vi "BotSpeak_Variables.vi"(1 "Scaling":T1(array[cluster])=[{"upper limit"=0.0, "lower limit"=0.0, "scale"=1.0}, {"upper limit"=0.0, "lower limit"=0.0, "scale"=1.0}, {"upper limit"=0.0, "lower limit"=0.0, "scale"=1.0}, {"upper limit"=0.0, "lower limit"=0.0, "scale"=1.0}, {"upper limit"=0.0, "lower limit"=0.0, "scale"=1.0}, {"upper limit"=0.0, "lower limit"=0.0, "scale"=1.0}, {"upper limit"=0.0, "lower limit"=0.0, "scale"=1.0}, {"upper limit"=0.0, "lower limit"=0.0, "scale"=1.0}, {"upper limit"=0.0, "lower limit"=0.0, "scale"=1.0}, {"upper limit"=0.0, "lower limit"=0.0, "scale"=1.0}, {"upper limit"=0.0, "lower limit"=0.0, "scale"=1.0}], 2 "Var #?":bool[](array[boolean])=[TRUE, TRUE, TRUE, TRUE, TRUE, TRUE, TRUE, TRUE, TRUE, TRUE, TRUE], 3 "Variables":string[](array[string])) -> (0 "Binary out":u8[](array[numeric]) format="%.0x")   [LabVIEW 2014]
panel:
  out "Vars":string[](array[string])
  # "Variable # or Value of Variable"
  # "sources:\n\n200 (C8) - TMR[#]\n201 (C9) - AI[#]\n202 (CA) - DIO[#]\n203 (CB) - PWM[#]\n204 (CC) - SERVO[#]\n205 (CD) - VAR[#]\n\n220 (DC) - TMR[var]\n221 (DD) - AI[var]\n222 (DE) - DIO[var]\n223 (DF) - PWM[var]\n224 (E0) - SERVO[var]\n225 (E1) - VAR[var]\n\n252 (FC) - \n253 (FD) - var[var]\n254 (FE) - \n255 (FF) - var#"
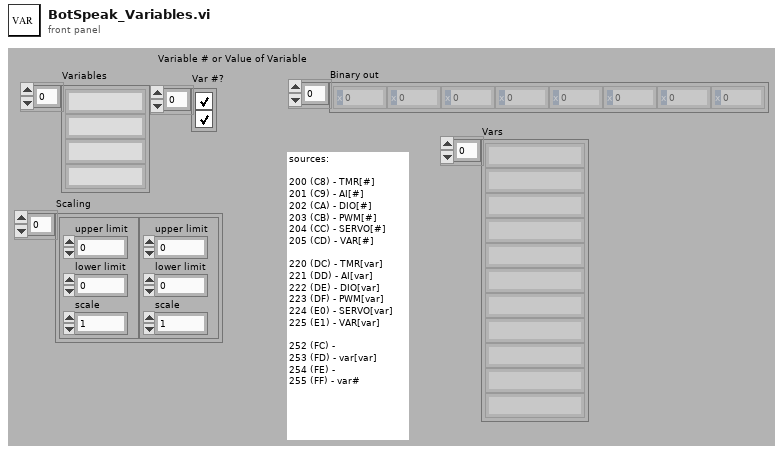
[diagram p1: front panel]
types:
  T1 = cluster{"upper limit":dbl, "lower limit":dbl, "scale":dbl}[]
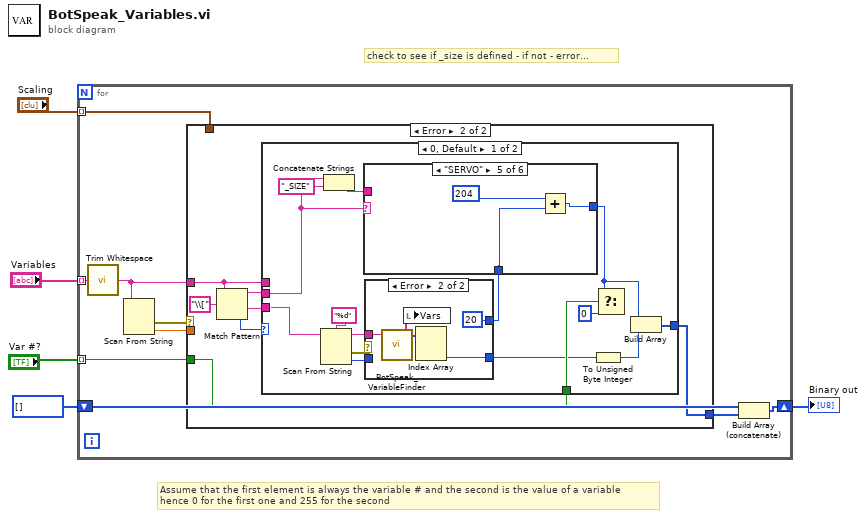
[diagram p0: block diagram]
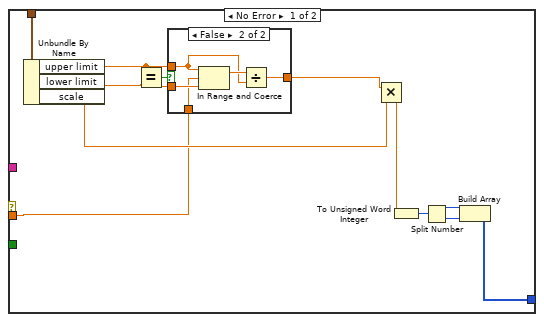
[diagram p2: hidden frame]
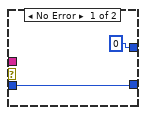
[diagram p4: hidden frame]
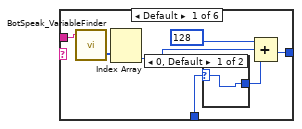
[diagram p5: hidden frame]
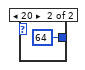
[diagram p6: hidden frame]
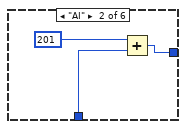
[diagram p7: hidden frame]
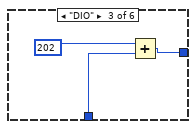
[diagram p8: hidden frame]
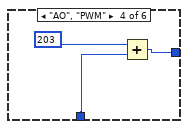
[diagram p9: hidden frame]
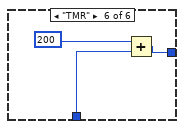
[diagram p10: hidden frame]
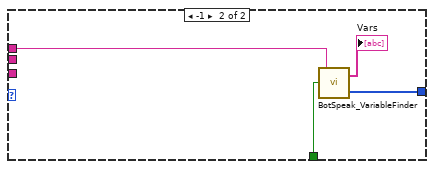
[diagram p11: hidden frame]
diagram:
  # "check to see if _size is defined - if not - error..."
  # "Assume that the first element is always the variable # and the second is the value of a variable\nhence 0 for the first one and 255 for the second"
  n1 = for {
    tunnel: "Variables" -> [w14] mode=indexing
    shift-right: [w11] -> w3
    shift-left: u8[] [] -> [w10]
    tunnel: "Scaling" -> [w8] mode=indexing
    tunnel: "Var #?" -> [w7] mode=indexing
    n2 = call <vilib>:"Trim Whitespace.vi"("string"=w14) -> ("trimmed string"=w6:string)  [unwired: 1 in]
    n3 = Scan From String(input string=w6) -> (error out=w13:errorcluster, output 1=w12:dbl)  [unwired: 4 in, 2 out]
    n4 = case shown="Error" w13 {
      tunnel: w6 -> [_ w38]
      tunnel: [w23 w35] -> w9
      tunnel: w12 -> [w15 _]
      tunnel: w8 -> [w22 _]
      tunnel: w7 -> [_ w34]
      frame No Error {
        n5 = Unbundle By Name(w22) -> ("upper limit"=w21:dbl, "lower limit"=w20:dbl, "scale"=w17:dbl)
        n6 = Equal?(x=w21, y=w20) -> (x = y?=w19:bool)
        n7 = case shown="False" w19 {
          tunnel: w20 -> [_ w31]
          tunnel: w21 -> [_ w30]
          tunnel: w15 -> [w27 w29]
          tunnel: [w27 w28] -> w18
          frame True {
          }
          frame False {
            n8 = In Range and Coerce(upper limit=w30, x=w29, lower limit=w31) -> (coerced(x)=w32:dbl)  [unwired: 1 out]
            n9 = Divide(x=w32, y=w30) -> (x/y=w28:dbl)
          }
        }
        n10 = Multiply(x=w18, y=w17) -> (x*y=w16:dbl)
        n11 = To Unsigned Word Integer(number=w16) -> (unsigned 16bit integer=w26:u16)
        n12 = Split Number(x=w26) -> (hi(x)=w25:u8, lo(x)=w24:u8)
        n13 = Build Array(w25, w24) -> (w23:u8[])
      }
      frame Error {
        n14 = Match Pattern(string=w38, regular expression="\\[" ("format string")) -> (before substring=w36:string, after substring=w33:string, offset past match=w39:i32)  [unwired: 1 in, 1 out]
        n15 = case shown="0, Default" w39 {
          tunnel: w38 -> [_ w88]
          tunnel: w33 -> [w45 _]
          tunnel: w36 -> [w44 _]
          tunnel: w34 -> [w50 w87]
          tunnel: [w49 w86] -> w35
          frame 0, Default {
            n16 = Scan From String(format string="%d", input string=w45) -> (error out=w48:errorcluster, output 1=w46:i32)  [unwired: 3 in, 2 out]
            n17 = Concatenate Strings(w44, "_SIZE" ("string")) -> (w42:string)
            n18 = case shown="Error" w48 {
              tunnel: [w55 w58] -> w47
              tunnel: w46 -> [w55 _]
              tunnel: w45 -> [_ w60]
              tunnel: [u8 0 ("element") u8 20 ("element")] -> w41
              frame No Error {
              }
              frame Error {
                n19 = call <userlib>:"BotSpeak_VariableFinder.vi"("variable name"=w60) -> ("codes"=w59:u8[], "Variables"=w56:string[])  [unwired: 2 in]
                n20 = local write "Vars"(w56) -> ()
                n21 = Index Array(array=w59) -> (element #2=w58:u8)  [unwired: 2 in, 1 out]
              }
            }
            n22 = case shown="\"SERVO\"" w44 {
              tunnel: [w64 w70 w73 w76 w79 w83] -> w40
              tunnel: w42 -> [w67 _ _ _ _ _]
              tunnel: w41 -> [w62 w71 w74 w77 w80 w84]
              frame Default {
                n23 = call <userlib>:"BotSpeak_VariableFinder.vi"("variable name"=w67) -> ("codes"=w66:u8[])  [unwired: 2 in, 1 out]
                n24 = Index Array(array=w66) -> (element #2=w63:u8)  [unwired: 2 in, 1 out]
                n25 = case shown="0, Default" w62 {
                  selector: w62 -> [w68 _]
                  tunnel: [w68 u8 64 ("element")] -> w61
                  frame 0, Default {
                  }
                  frame 20 {
                  }
                }
                n26 = Compound Arithmetic op=ADD(u8 128 ("element"), w63, w61) -> (w64:u8)
              }
              frame "AI" {
                n27 = Add(x=u8 201 ("element"), y=w71) -> (x+y=w70:u8)
              }
              frame "DIO" {
                n28 = Add(x=u8 202 ("element"), y=w74) -> (x+y=w73:u8)
              }
              frame "AO", "PWM" {
                n29 = Add(x=u8 203 ("element"), y=w77) -> (x+y=w76:u8)
              }
              frame "SERVO" {
                n30 = Add(x=u8 204 ("element"), y=w80) -> (x+y=w79:u8)
              }
              frame "TMR" {
                n31 = Add(x=u8 200 ("element"), y=w84) -> (x+y=w83:u8)
              }
            }
            n32 = To Unsigned Byte Integer(number=w47) -> (unsigned 8bit integer=w51:u8)
            n33 = Select(t=w40, s=w50, f=u8 0 ("element")) -> ()  [unwired: 1 out]
            n34 = Build Array(w40, w51) -> (w49:u8[])
          }
          frame -1 {
            n35 = call <userlib>:"BotSpeak_VariableFinder.vi"("Var #?"=w87, "variable name"=w88) -> ("codes"=w86:u8[], "Variables"=→"Vars":string[])  [unwired: 1 in]
          }
        }
      }
    }
    n36 = Build Array (concatenate)(w10, w9) -> (w11:u8[])
  }
  "Binary out" <- w3
